vi "Check_Beam_Powers.vi"(3 "Mode":T6, 5 "Traverse line In":T3 {"Row Duration (mins)" format="%#.1f"; "Row No" min=0; "Trace Gas Concentration (%)" min=0.0 format="%#.2f"; "Emission Rate (l/min)" format="%#.2f"; "Tunnel Speed" format="%#.2f"; "Start X" format="%#.2f"; "Start Y" format="%#.2f"; "Start Z" format="%#.2f"; "End X" format="%#.2f"; "End Y" format="%#.2f"; "End Z" format="%#.2f"; "Averaging time (min)" min=0.0 format="%#.1f"}) -> (0 "Error Message":string, 1 "Status":T2, 2 "Traverse line Out":T3 {"Row Duration (mins)" format="%#.1f"; "Row No" min=0; "Trace Gas Concentration (%)" min=0.0 format="%#.2f"; "Emission Rate (l/min)" format="%#.2f"; "Tunnel Speed" format="%#.2f"; "Start X" format="%#.2f"; "Start Y" format="%#.2f"; "Start Z" format="%#.2f"; "End X" format="%#.2f"; "End Y" format="%#.2f"; "End Z" format="%#.2f"; "Averaging time (min)" min=0.0 format="%#.1f"})   [LabVIEW 2010]
uses:
  Gen Trav/Traverse_cluster.ctl
  Gen Trav/Spacing.ctl
  Controls/Multi_run_mode.ctl
  Controls/User_Specific_mode.ctl
  Gen Trav/Multi_Run_Status.ctl
  Controls/Beam_Type.ctl
  ADAM Client/Sub VIs/ADAM Controls/Remember_value_mode.ctl
  Gen Trav/Route mapping/Axis.ctl
  Controls/Save_Data.ctl
  Controls/Setup.ctl
  Globals/Meas_global.vi
  Globals/Constants_global.vi
  Globals/LDA_meas_global_1.vi
  Globals/LDA_meas_global_2.vi
panel:
  out "Light Power":dbl=8.10606551e-08 format="%^#_9e"
  in  "stop":bool
  out "Poor Beam Power?":bool
  in  "Update Datum Powers?":bool
  out "Powers":dbl[](array[numeric]) format="%.4f"
  out "Beam Data":dbl[][](array[numeric]) format="%.4f"
  out "Beam Type":T1 items=["Green Unshifted", "Green Shifted", "Blue Unshifted", "Blue Shifted"]
  # "X                      Y                   Z          Datum Power"
  # "Green Unshifted\nGreen Shifted\nBlue Unshifted\nBlue Shifted"
  # "X           Y            Z"
  # "Start"
  # "End"
  # "X           Y            Z"
  # "Start"
  # "End"
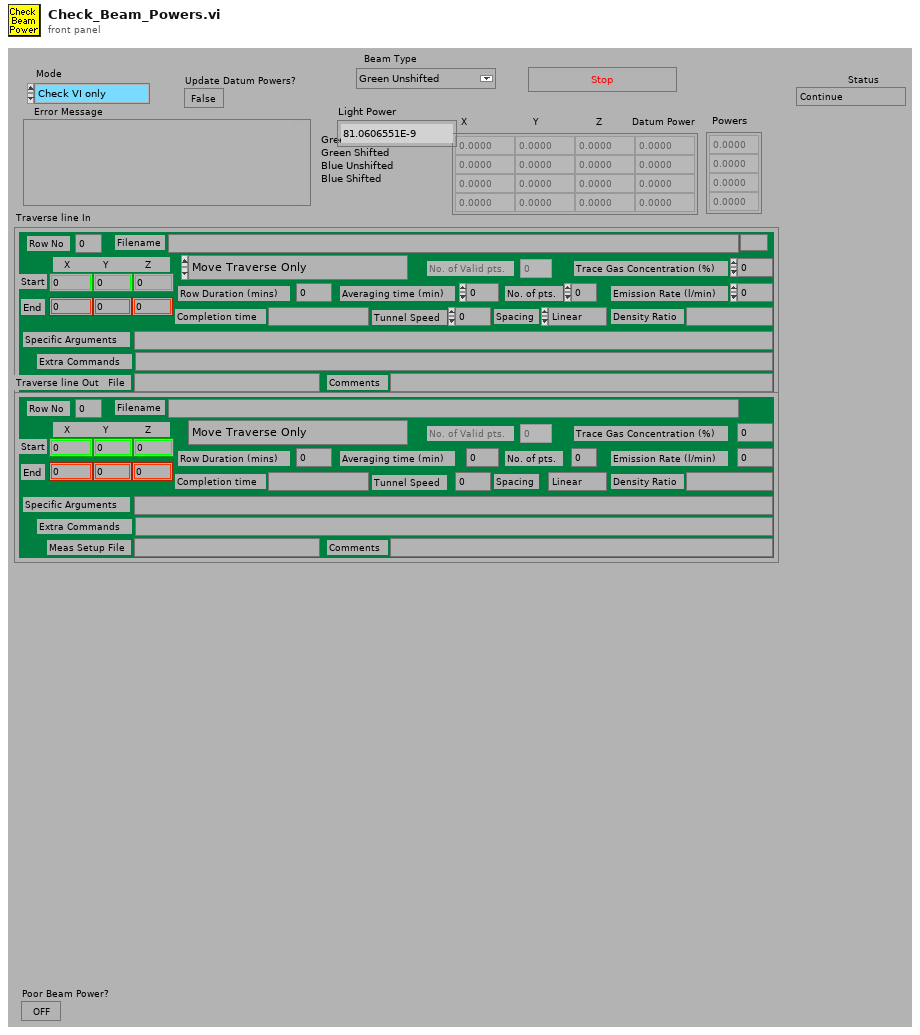
[diagram p1: front panel]
types:
  T1 = typedef "Beam_Type.ctl" = u16
  T2 = typedef "Multi_Run_Status.ctl" = enum16{"Continue", "Jump to Next Point", "Jump to Next Row", "Jump To Fall Back", "Terminate Run"}
  T3 = typedef "Traverse_cluster.ctl" = cluster{"Start X":dbl, "Start Y":dbl, "Start Z":dbl, "End X":dbl, "End Y":dbl, "End Z":dbl, "No. of pts.":i32, "Spacing":T4, "Filename":path, "Tunnel Speed":dbl, "Averaging time (min)":dbl, "Extra Commands":string, "Specific Arguments":string, "Emission Rate (l/min)":dbl, "Trace Gas Concentration (%)":dbl, "Density Ratio":string, "Comments":string, "Row No":i32, "Row Type Selector":T5, "Completion time":string, "Row Duration (mins)":dbl, "No. of Valid pts.":i32, "Meas Setup File":string}
  T4 = typedef "Spacing.ctl" = enum16{"Linear", "Log", "Gauss", "Specified", "N/A"}
  T5 = typedef "Multi_run_mode.ctl" = enum16{"Move Traverse Only", "Set Tunnel Speed Only", "Set Source Only", "Set Measurement Conditions", "Single Measurement", "Vertical Profile", "Lateral Profile", "Longitudinal Profile", "Explore Volume", "Multi-Axis Profile", "Auto Calibrate", "Meas Fast FID Bkgnd", "Check Beam Power", "Scanning Valve Measurement", "Run VI Named:", "Set ADAM Ch", "Wait (minutes)", "Send Message", "Synchronize With:", "Fall Back to this Row", "Turn Off Row Repeating", "Blank Row"}
  T6 = typedef "User_Specific_mode.ctl" = enum16{"Check VI only", "Run VI"}
  T7 = enum32{"Bad", "Idle", "Run top level", "Running"}
  T8 = enum16{"Load From Excel File", "Save to Excel File"}
  T9 = typedef "Remember_value_mode.ctl" = enum16{"Read only", "Read and Write"}
  T10 = typedef "Axis.ctl" = enum16{"X Axis", "X Axis -ve", "Y Axis", "Y Axis -ve", "Z Axis", "Z Axis -ve"}
  T11 = typedef "Save_Data.ctl" = enum16{"Save No Data", "Save Data"}
  T12 = typedef "Setup.ctl" = enum16{"Run Program", "Show Setup", "Save Current Setup", "Setup Front Panel"}
  T13 = typedef "Status_Cluster.ctl" = cluster{"Status":T2, "Error Type":string, "Error Description":string}
  T14 = typedef "BSA_Type.ctl" = enum16{"57N11", "BSA F60"}
  T15 = typedef "BSA_info_Cluster.ctl" = cluster{"GPIB Address":string, "No of Check Bytes":i32, "Extra Info":string, "COLOUR":u32, "Wavelength (nm)":dbl}
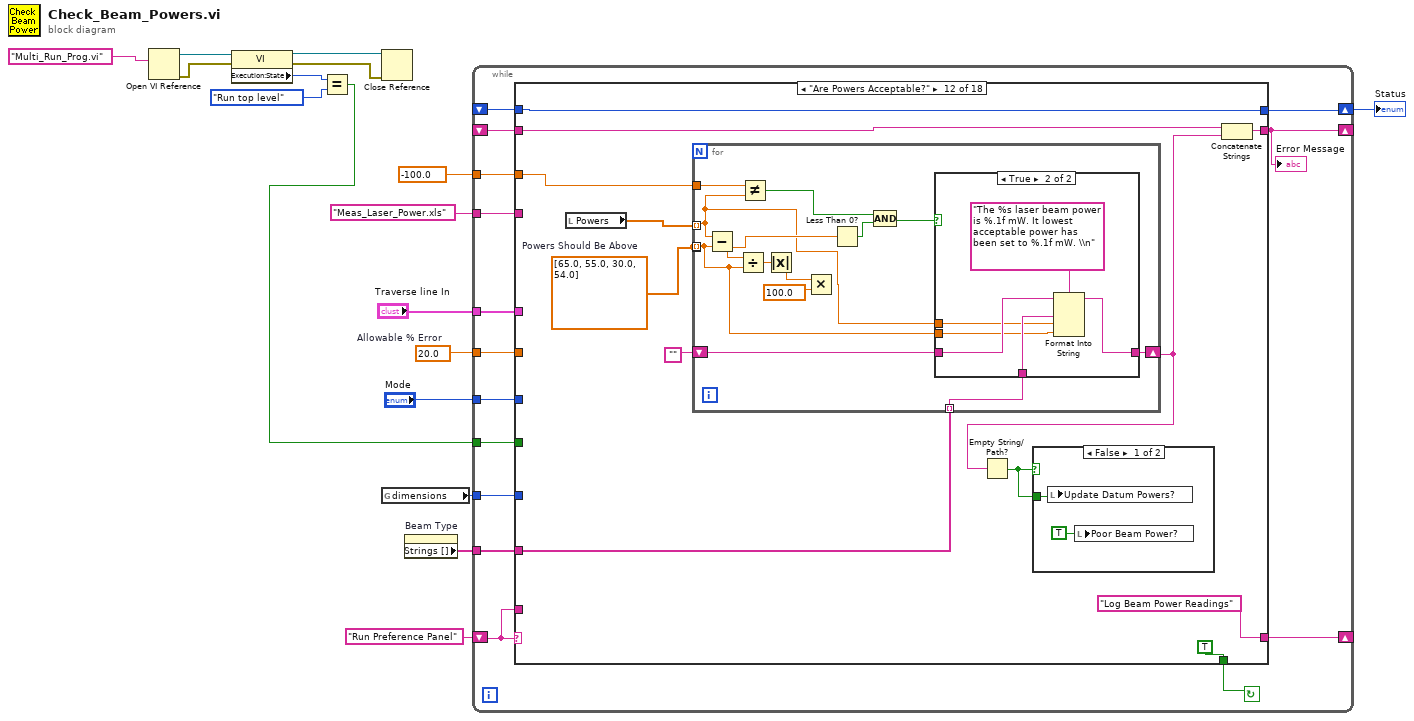
[diagram p0: block diagram]
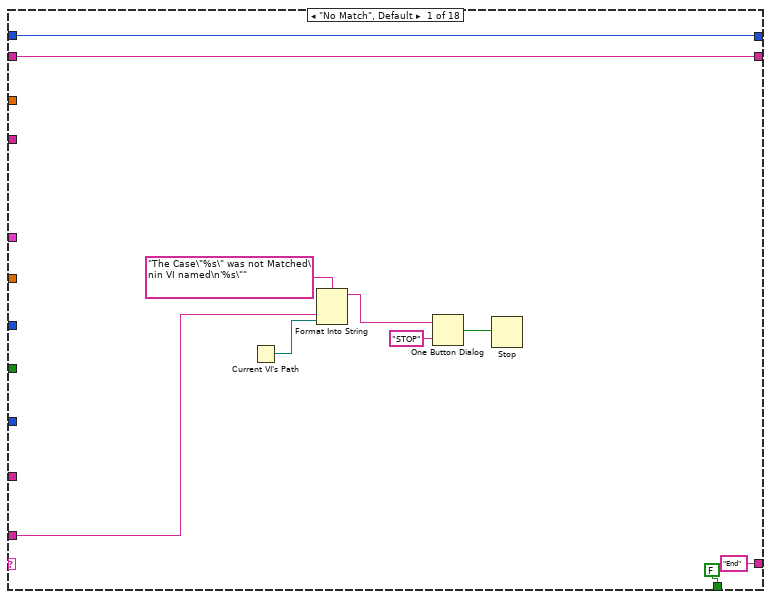
[diagram p2: hidden frame]
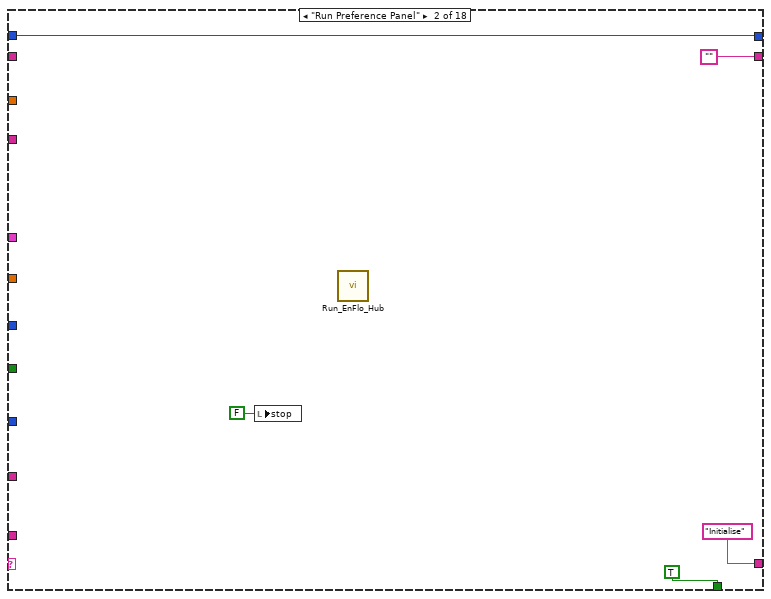
[diagram p3: hidden frame]
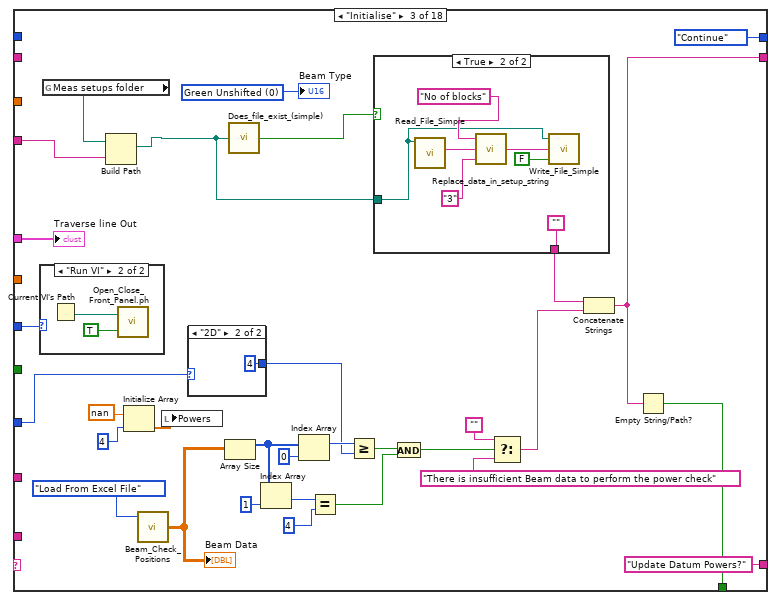
[diagram p4: hidden frame]
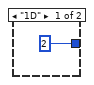
[diagram p5: hidden frame]
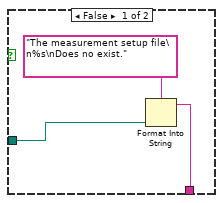
[diagram p6: hidden frame]
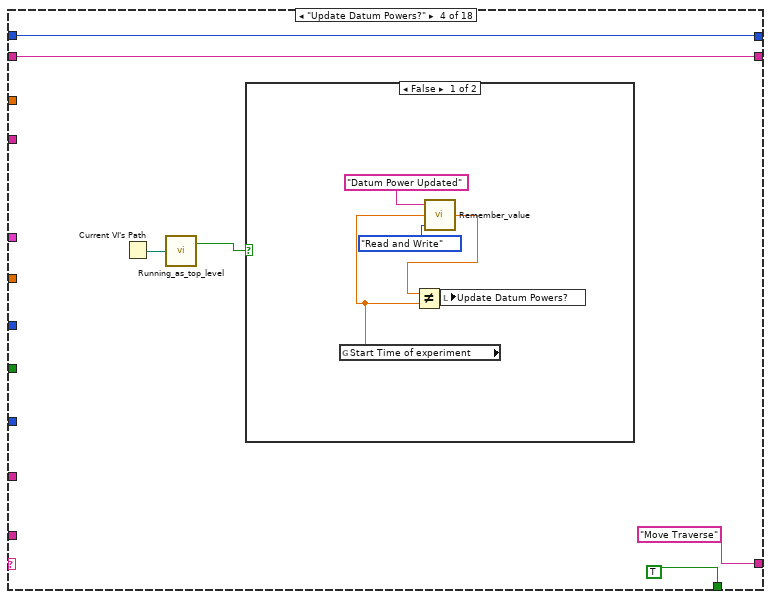
[diagram p8: hidden frame]
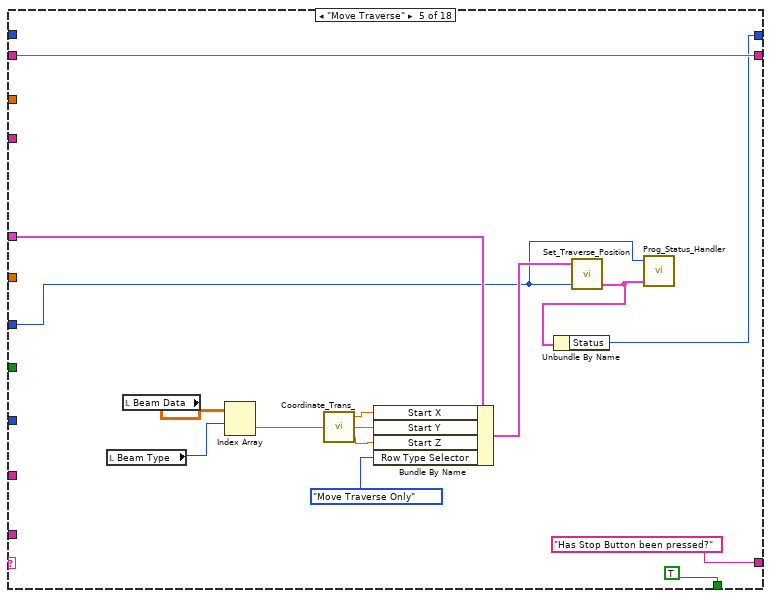
[diagram p10: hidden frame]
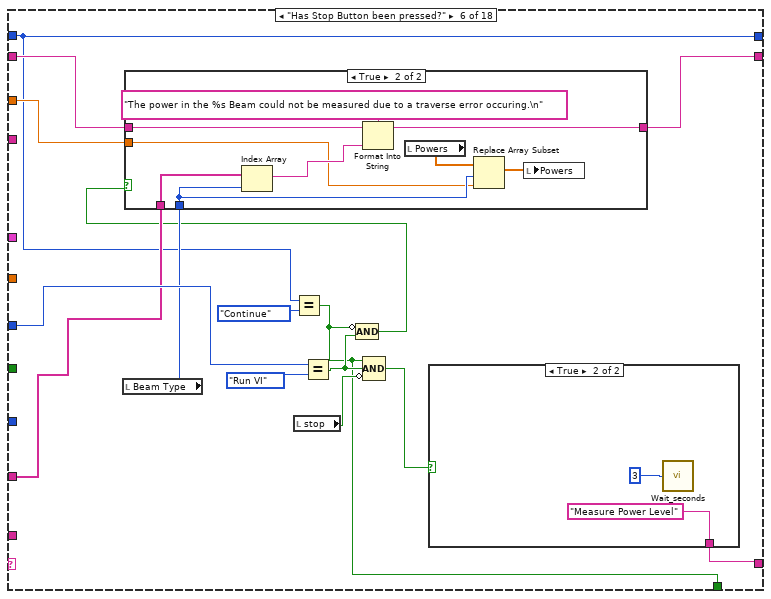
[diagram p11: hidden frame]
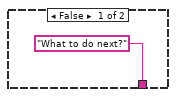
[diagram p13: hidden frame]
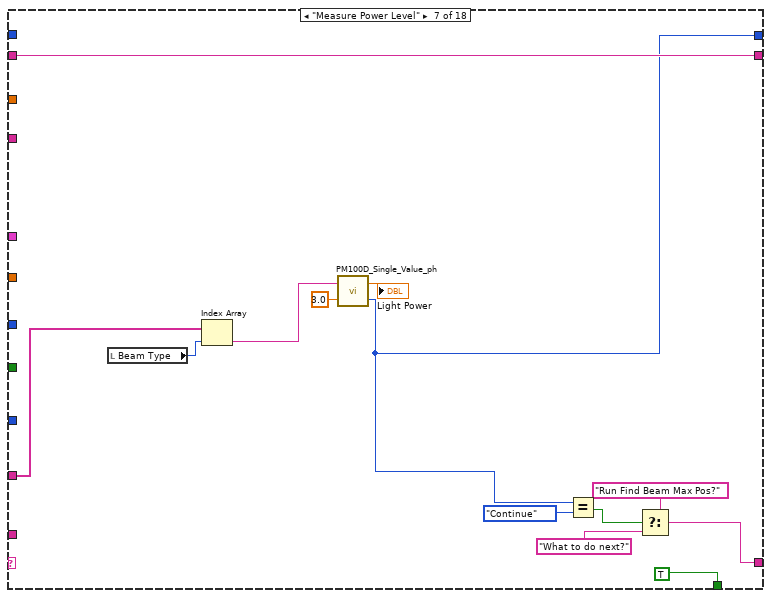
[diagram p14: hidden frame]
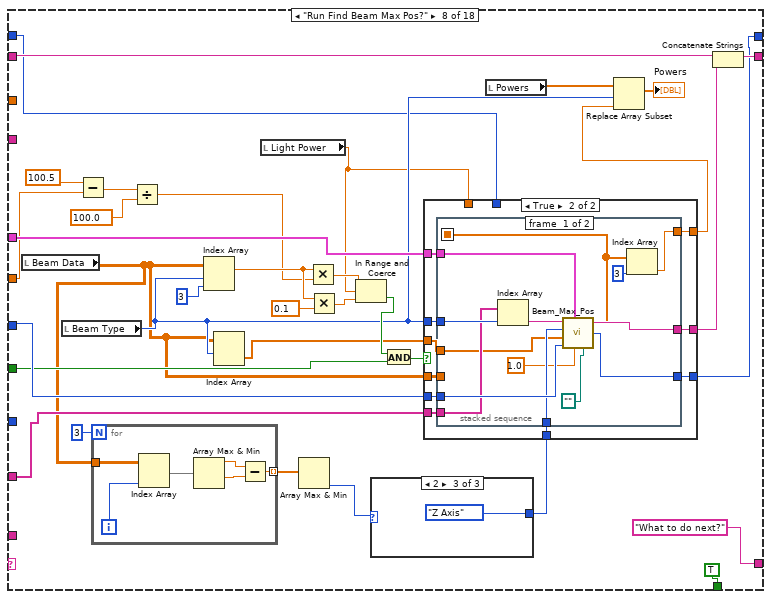
[diagram p15: hidden frame]
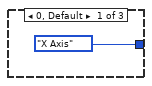
[diagram p16: hidden frame]
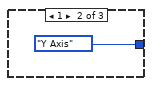
[diagram p17: hidden frame]
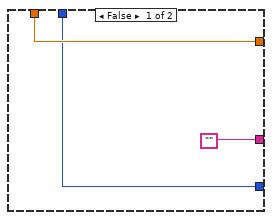
[diagram p18: hidden frame]
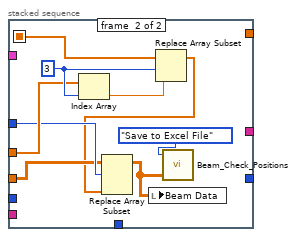
[diagram p19: hidden frame]
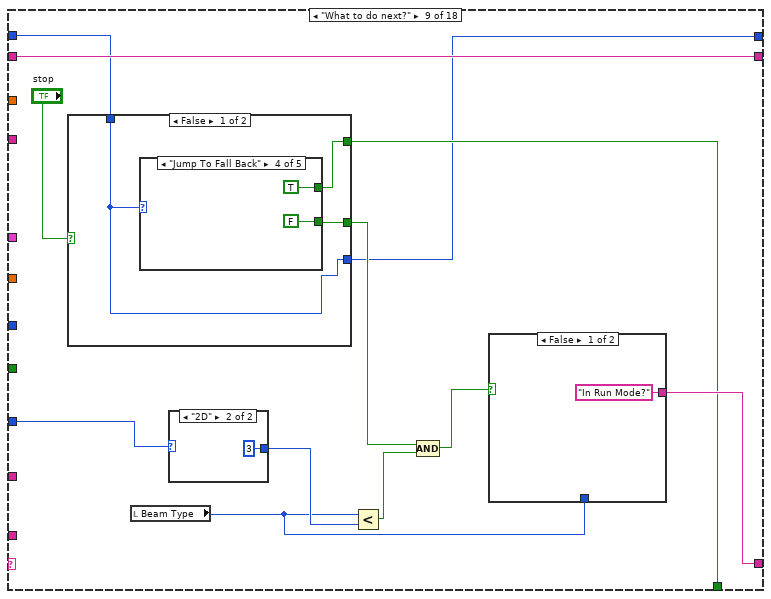
[diagram p20: hidden frame]
diagram:
  w12 = 20.0  # Allowable % Error
  n1 = Open VI Reference(vi path="Multi_Run_Prog.vi") -> (vi reference=w6:refnum<vi>, error out=w7:errorcluster)  [unwired: 1 in, 4 out]
  n2 = property class="VI"(reference=w6, error in=w7) -> (reference out=w8:refnum<vi>, error out=w9:errorcluster, "Execution:State"=w5:T7)
  n3 = Equal?(x=w5, y=T7."Run top level" ("Exec.State")) -> (x = y?=w3:bool)
  n4 = Close Reference(reference=w8, error in (no error)=w9) -> ()  [unwired: 1 out]
  n5 = global read "Meas_global.vi" "dimensions"() -> (w14:enum16{"1D", "2D"})
  n6 = property on="Beam Type" class="Ring (strict)"() -> ("Strings []"=w15:string[])  [unwired: 2 in, 2 out]
  n7 = while {
    tunnel: -100.0 ("Element Data") -> [w21]
    tunnel: w12 -> [w23]
    shift-left: _ -> [w25]
    shift-right: [w24] -> _
    tunnel: "Meas_Laser_Power.xls" -> [w26]
    tunnel: w14 -> [w27]
    tunnel: w15 -> [w30]
    tunnel: "Traverse line In" -> [w31]
    tunnel: "Mode" -> [w32]
    shift-left: "Run Preference Panel" -> [w22]
    shift-right: [w28] -> _
    tunnel: w3 -> [w20]
    shift-right: [w19] -> w1
    shift-left: _ -> [w18]
    stop <- w29 continue-if-true
    n8 = case shown="\"Are Powers Acceptable?\"" w22 {
      tunnel: w31 -> [_ _ w73 _ w118 _ _ w192 _ _ _ _ _ _ _ _ w441 _]
      tunnel: w32 -> [_ _ w70 _ w113 w131 _ w191 _ w280 _ _ _ _ _ _ w445 w450]
      tunnel: w30 -> [_ _ _ _ _ w129 w149 w166 _ _ w293 w335 _ _ _ _ _ _]
      tunnel: [FALSE ("Update Datum Powers?") TRUE ("Update Datum Powers?") w62 TRUE ("Update Datum Powers?") TRUE w120 TRUE TRUE w241 TRUE ("Update Datum Powers?") TRUE TRUE TRUE TRUE ("Update Datum Powers?") TRUE ("Update Datum Powers?") w411 w442 FALSE ("Update Datum Powers?")] -> w29
      tunnel: ["End" "Initialise" "Update Datum Powers?" "Move Traverse" "Has Stop Button been pressed?" w130 w154 "What to do next?" w243 w275 "Are Powers Acceptable?" "Log Beam Power Readings" w362 "Update Datum Powers and Positions" "Take datum velocity measurement?" "Move traverse to datum location" "Take a datum velocity measurement" "End"] -> w28
      tunnel: w27 -> [_ _ w69 _ _ _ _ _ w249 _ _ _ _ _ _ w413 _ _]
      tunnel: w26 -> [_ _ w75 _ _ _ _ _ _ _ _ _ _ _ _ _ _ _]
      tunnel: w25 -> [w34 _ _ w95 w111 w127 w156 w178 w245 w279 w291 w333 w363 w388 w398 w415 w447 w453]
      tunnel: [w34 "" w50 w95 w111 w128 w156 w177 w245 w279 w290 w332 w364 "" w398 w415 w447 w453] -> w24
      tunnel: w23 -> [_ _ _ _ _ _ _ w174 _ _ w286 _ _ _ _ _ _ _]
      tunnel: w22 -> [w37 _ _ _ _ _ _ _ _ _ _ _ _ _ _ _ _ _]
      tunnel: w21 -> [_ _ _ _ _ w126 _ _ _ _ w283 w327 _ _ _ _ _ _]
      tunnel: w20 -> [_ _ _ _ _ _ _ w167 _ _ _ _ _ _ _ w410 _ _]
      tunnel: [w33 w43 Multi_Run_Status."Continue" ("Status") w93 w104 w119 w151 w161 w239 w273 w282 w326 w360 w384 w394 w408 w440 w449] -> w19
      tunnel: w18 -> [w33 w43 _ w93 _ w119 _ w160 w240 w273 w282 w326 w360 w384 w394 w408 _ w448]
      frame "No Match", Default {
        n9 = Current VI's Path() -> (path=w38:path)
        n10 = Format Into String(format string="The Case\"%s\" was not Matched\nin VI named\n'%s\"" ("Format String"), w37, w38) -> (resulting string=w41:string)  [unwired: 2 in, 1 out]
        n11 = One Button Dialog(message=w41, button name ("OK")="STOP") -> (true=w39:bool)
        n12 = Stop(stop? (T)=w39) -> ()
      }
      frame "Run Preference Panel" {
        n13 = local write "stop"(FALSE ("stop")) -> ()
        n14 = call "Run_EnFlo_Hub.vi"() -> ()  [unwired: 8 out]
      }
      frame "Initialise" {
        w77 = T1 0 items=["Green Unshifted", "Green Shifted", "Blue Unshifted", "Blue Shifted"] ("Beam Type")
        n15 = case shown="\"Run VI\"" w70 {
          frame "Check VI only" {
          }
          frame "Run VI" {
            n16 = Current VI's Path() -> (path=w91:path)
            n17 = call "Open_Close_Front_Panel.ph.vi"("Front Panel Window:Open"=TRUE, "VI path"=w91) -> ()  [unwired: 2 out]
          }
        }
        n18 = global read "Constants_global.vi" "Meas setups folder"() -> (w76:path)
        n19 = Build Path(base path=w76, name or relative path=w75) -> (appended path=w51:path)
        n20 = Initialize Array(nan ("Numeric"), 4 ("Dimension Size")) -> (w52:dbl[])
        n21 = call "Beam_Check_Positions.vi"("Mode"=T8."Load From Excel File") -> ("Values Out"=w72:dbl[][])  [unwired: 1 in, 1 out]
        "Beam Data" <- w72
        n22 = local write "Powers"(w52) -> ()
        n23 = case shown="\"2D\"" w69 {
          tunnel: [2 4] -> w67
          frame "1D" {
          }
          frame "2D" {
          }
        }
        n24 = Array Size(array=w72) -> (size(s)=w60:i32[])
        n25 = call "Does_file_exist_(simple).vi"("Pathname"=w51) -> ("exists?"=w74:bool)
        n26 = Index Array(array=w60, index=1 ("Index")) -> (element=w59:i32)
        n27 = Index Array(array=w60, index=0 ("Index")) -> (element=w68:i32)
        n28 = Equal?(x=w59, y=4) -> (x = y?=w56:bool)
        n29 = Greater Or Equal?(x=w68, y=w67) -> (x >= y?=w57:bool)
        n30 = case shown="True" w74 {
          tunnel: w51 -> [w83 w84]
          tunnel: [w81 ""] -> w64
          frame False {
            n31 = Format Into String(format string="The measurement setup file\n%s\nDoes no exist." ("Format String"), w83) -> (resulting string=w81:string)  [unwired: 2 in, 1 out]
          }
          frame True {
            n32 = call "Read_File_Simple.vi"("Filename"=w84) -> ("string"=w89:string)  [unwired: 2 in, 7 out]
            n33 = call "Replace_data_in_setup_string.vi"("New data string"="3", "Input string"=w89, "Variable name"="No of blocks") -> ("Appended string"=w86:string)
            n34 = call "Write_File_Simple.vi"("append to file? (new file:F)"=FALSE, "character string"=w86, "file path"=w84) -> ()  [unwired: 2 out]
          }
        }
        n35 = And(x=w57, y=w56) -> (x .and. y?=w55:bool)
        n36 = Select(t="", s=w55, f="There is insufficient Beam data to perform the power check") -> (s? t:f=w63:string)
        n37 = Concatenate Strings(w64, w63) -> (w50:string)
        n38 = Empty String/Path?(string/path=w50) -> (empty?=w62:bool)
        "Beam Type" <- w77
        "Traverse line Out" <- w73
      }
      frame "Update Datum Powers?" {
        n39 = Current VI's Path() -> (path=w97:path)
        n40 = call "Running_as_top_level.vi"("Vi path name"=w97) -> ("Top Level"=w96:bool)  [unwired: 1 out]
        n41 = case shown="False" w96 {
          frame False {
            n42 = global read "Meas_global.vi" "Start Time of experiment"() -> (w101:dbl)
            n43 = call "Remember_value.vi"("Mode"=Remember_value_mode."Read and Write", "Input Value"=w101, "Ch name"="Datum Power Updated") -> ("Output Value"=w102:dbl)
            n44 = Not Equal?(x=w102, y=w101) -> (x != y?=w99:bool)
            n45 = local write "Update Datum Powers?"(w99) -> ()
          }
          frame True {
          }
        }
      }
      frame "Move Traverse" {
        n46 = local read "Beam Type"() -> (w109:T1)
        n47 = local read "Beam Data"() -> (w110:dbl[][])
        n48 = Index Array(array=w110, index (row)=w109) -> (element=w105:dbl[])  [unwired: 1 in]
        n49 = call "Coordinate_Trans_.vi"("Input Position"=w105) -> ("X"=w108:dbl, "Y"=w107:dbl, "Z"=w106:dbl)
        n50 = Bundle By Name(cluster=w118, "Start X"=w108, "Start Y"=w107, "Start Z"=w106, "Row Type Selector"=Multi_run_mode."Move Traverse Only") -> (w116:T3)
        n51 = call "Set_Traverse_Position.vi"("Simulate/Run"=w113, "Traverse line"=w116) -> ("Status Cluster"=w114:T13)  [unwired: 1 in, 2 out]
        n52 = Unbundle By Name(w114) -> ("Status"=w104:T2)
        n53 = call "Prog_Status_Handler.vi"("Status Cluster"=w114, "Simulate/Run"=w113) -> ()  [unwired: 2 out]
      }
      frame "Has Stop Button been pressed?" {
        n54 = local read "Beam Type"() -> (w125:T1)
        n55 = Equal?(x=w119, y=Multi_Run_Status."Continue" ("Status")) -> (x = y?=w120:bool)
        n56 = local read "stop"() -> (w124:bool)
        n57 = Equal?(x=w131, y=User_Specific_mode."Run VI" ("Mode")) -> (x = y?=w122:bool)
        n58 = Compound Arithmetic op=AND(invert w120, w122) -> (w121:bool)
        n59 = case shown="True" w121 {
          tunnel: w125 -> [_ w136]
          tunnel: w129 -> [_ w143]
          tunnel: w127 -> [w134 w140]
          tunnel: [w134 w139] -> w128
          tunnel: w126 -> [_ w135]
          frame False {
          }
          frame True {
            n60 = Index Array(array=w143, index=w136) -> (element=w142:string)
            n61 = Format Into String(format string="The power in the %s Beam could not be measured due to a traverse error occuring.\n" ("Format String"), initial string=w140, w142) -> (resulting string=w139:string)  [unwired: 1 in, 1 out]
            n62 = local read "Powers"() -> (w138:dbl[])
            n63 = Replace Array Subset(array=w138, new element=w135, index=w136) -> (w137:dbl[])
            n64 = local write "Powers"(w137) -> ()
          }
        }
        n65 = Compound Arithmetic op=AND(w120, w122, invert w124) -> (w123:bool)
        n66 = case shown="True" w123 {
          tunnel: ["What to do next?" "Measure Power Level"] -> w130
          frame False {
          }
          frame True {
            n67 = call "Wait_seconds.vi"("Seconds to wait"=u32 3) -> ()
          }
        }
      }
      frame "Measure Power Level" {
        n68 = local read "Beam Type"() -> (w150:T1)
        n69 = Index Array(array=w149, index=w150) -> (element=w148:string)
        n70 = call "PM100D_Single_Value_ph.vi"("Averaging Period (s)"=3.0, "Beam Name"=w148) -> ("Status"=w151:T2, "Light Power mW"=→"Light Power":dbl)
        n71 = Equal?(x=w151, y=Multi_Run_Status."Continue" ("Status")) -> (x = y?=w157:bool)
        n72 = Select(t="Run Find Beam Max Pos?", s=w157, f="What to do next?") -> (s? t:f=w154:string)
      }
      frame "Run Find Beam Max Pos?" {
        n73 = local read "Beam Data"() -> (w163:dbl[][])
        n74 = local read "Beam Type"() -> (w165:T1)
        n75 = Subtract(x=100.5, y=w174) -> (x-y=w173:dbl)
        n76 = for {
          N: 3 -> [_]
          tunnel: w163 -> [w201]
          tunnel: [w197] -> w189 mode=indexing
          i -> [w202]
          n77 = Index Array(array=w201, index (col)=w202) -> (element=w200:dbl[])  [unwired: 1 in]
          n78 = Array Max & Min(array=w200) -> (max value=w199:dbl, min value=w198:dbl)  [unwired: 2 out]
          n79 = Subtract(x=w199, y=w198) -> (x-y=w197:dbl)
        }
        n80 = Divide(x=w173, y=100.0) -> (x/y=w171:dbl)
        n81 = Index Array(array=w163, index (row)=w165, index (col)=3 ("Index")) -> (element=w185:dbl)
        n82 = Index Array(array=w163, index (row)=w165) -> (element=w164:dbl[])  [unwired: 1 in]
        n83 = local read "Light Power"() -> (w162:dbl)
        n84 = Array Max & Min(array=w189) -> (min index (indices)=w188:i32)  [unwired: 3 out]
        n85 = Multiply(x=w185, y=w171) -> (x*y=w183:dbl)
        n86 = Multiply(x=w185, y=0.1) -> (x*y=w182:dbl)
        n87 = In Range and Coerce(upper limit=w183, x=w162, lower limit=w182) -> (In Range?=w169:bool)  [unwired: 1 out]
        n88 = case shown="2" w188 {
          tunnel: [Axis."X Axis" ("Fixed Axis") Axis."Y Axis" ("Fixed Axis") Axis."Z Axis" ("Fixed Axis")] -> w187
          frame 0, Default {
          }
          frame 1 {
          }
          frame 2 {
          }
        }
        n89 = And(x=w169, y=w167) -> (x .and. y?=w168:bool)
        n90 = case shown="True" w168 {
          tunnel: w165 -> [_ w210]
          tunnel: w192 -> [_ w215]
          tunnel: w191 -> [_ w214]
          tunnel: w187 -> [_ w213]
          tunnel: [w205 w212] -> w179
          tunnel: w162 -> [w205 _]
          tunnel: ["" w211] -> w176
          tunnel: w166 -> [_ w209]
          tunnel: w164 -> [_ w208]
          tunnel: w163 -> [_ w207]
          tunnel: [w203 w206] -> w161
          tunnel: w160 -> [w203 _]
          frame False {
          }
          frame True {
            n91 = stacked-sequence {
              seq-local: [w218 _] -> [_ w236]
              tunnel: w215 -> [w229 _]
              tunnel: w214 -> [w228 _]
              tunnel: w213 -> [w227 _]
              tunnel: [w225 _] -> w212
              tunnel: [w224 _] -> w211
              tunnel: w210 -> [w222 w234]
              tunnel: w209 -> [w221 _]
              tunnel: w208 -> [w219 w235]
              tunnel: w207 -> [_ w233]
              tunnel: [w216 _] -> w206
              frame #0 {
                n92 = Index Array(array=w221, index=w222) -> (element=w220:string)
                n93 = call "Beam_Max_Pos.vi"("Picture Log"=path "", "Search Step (mm)"=1.0, "Mode"=w228, "Starting Position"=w219, "Traverse line In"=w229, "Fixed Axis"=w227, "Beam Name"=w220) -> ("Status"=w216:T2, "Beam maxima"=w218:dbl[], "Message"=w224:string)  [unwired: 1 out]
                n94 = Index Array(array=w218, index=3 ("Index")) -> (element=w225:dbl)
              }
              frame #1 {
                w237 = 3 ("index")
                n95 = Index Array(array=w235, index=w237) -> (element=w238:dbl)
                n96 = Replace Array Subset(array=w236, new element=w238, index=w237) -> (w230:dbl[])
                n97 = Replace Array Subset(array=w233, new element=w230, index (row)=w234) -> (w232:dbl[][])  [unwired: 1 in]
                n98 = local write "Beam Data"(w232) -> ()
                n99 = call "Beam_Check_Positions.vi"("Values"=w232, "Mode"=T8."Save to Excel File") -> ()  [unwired: 2 out]
              }
            }
          }
        }
        n100 = local read "Powers"() -> (w181:dbl[])
        n101 = Replace Array Subset(array=w181, new element=w179, index=w165) -> (→"Powers":dbl[])
        n102 = Concatenate Strings(w178, w176) -> (w177:string)
      }
      frame "What to do next?" {
        n103 = case shown="False" "stop" {
          tunnel: [w253 FALSE] -> w242
          tunnel: [w252 FALSE] -> w241
          tunnel: w240 -> [w251 _]
          tunnel: [w251 Multi_Run_Status."Terminate Run" ("Status")] -> w239
          frame False {
            n104 = case shown="\"Jump To Fall Back\"" w251 {
              tunnel: [TRUE TRUE FALSE FALSE FALSE] -> w253
              tunnel: [TRUE TRUE TRUE TRUE FALSE] -> w252
              frame "Continue" {
              }
              frame "Jump to Next Point" {
              }
              frame "Jump to Next Row" {
              }
              frame "Jump To Fall Back" {
              }
              frame "Terminate Run" {
              }
            }
          }
          frame True {
          }
        }
        n105 = local read "Beam Type"() -> (w246:T1)
        n106 = case shown="\"2D\"" w249 {
          tunnel: [1 3] -> w250
          frame "1D" {
          }
          frame "2D" {
          }
        }
        n107 = Less?(x=w246, y=w250) -> (x < y?=w248:bool)
        n108 = Compound Arithmetic op=AND(w242, w248) -> (w247:bool)
        n109 = case shown="False" w247 {
          tunnel: w246 -> [_ w270]
          tunnel: ["In Run Mode?" "Move Traverse"] -> w243
          frame False {
          }
          frame True {
            n110 = Increment(x=w270) -> (x+1=w269:T1)
            n111 = local write "Beam Type"(w269) -> ()
          }
        }
      }
      frame "In Run Mode?" {
        n112 = Equal?(x=w280, y=User_Specific_mode."Run VI" ("Mode")) -> (x = y?=w277:bool)
        n113 = Select(t="Compare Powers with Datum values", s=w277, f="Move traverse to datum location") -> (s? t:f=w275:string)
      }
      frame "Compare Powers with Datum values" {
        n114 = local read "Beam Data"() -> (w296:dbl[][])
        n115 = local read "Powers"() -> (w295:dbl[])
        n116 = Index Array(array=w296, index (col)=3 ("Index")) -> (element=w294:dbl[])  [unwired: 1 in]
        n117 = for {
          tunnel: w295 -> [w301] mode=indexing
          tunnel: w294 -> [_] mode=indexing
          tunnel: w294 -> [w312] mode=indexing
          shift-right: [w316] -> w289
          shift-left: "" -> [w318]
          tunnel: w293 -> [w317] mode=indexing
          tunnel: "Update Datum Powers?" -> [w315]
          tunnel: w286 -> [w302]
          tunnel: w283 -> [w300]
          n118 = Subtract(x=w301, y=w312) -> (x-y=w310:dbl)
          n119 = Not Equal?(x=w300, y=w301) -> (x != y?=w299:bool)
          n120 = Divide(x=w310, y=w312) -> (x/y=w311:dbl)
          n121 = Greater Than 0?(x=w310) -> (x > 0?=w306:bool)
          n122 = Absolute Value(x=w311) -> (abs(x)=w309:dbl)
          n123 = Multiply(x=w309, y=100.0) -> (x*y=w307:dbl)
          n124 = Greater?(x=w307, y=w302) -> (0:w308:bool)
          n125 = Select(t="above", s=w306, f="below") -> (s? t:f=w303:string)
          n126 = Compound Arithmetic op=AND(w299, invert w315, w308) -> (w314:bool)
          n127 = case shown="True" w314 {
            tunnel: w318 -> [w319 w324]
            tunnel: w317 -> [_ w325]
            tunnel: [w319 w323] -> w316
            tunnel: w307 -> [_ w321]
            tunnel: w303 -> [_ w320]
            frame False {
            }
            frame True {
              n128 = Format Into String(format string="The %s laser beam is %.1f%% %s its datum value\\n" ("Format String"), initial string=w324, w325, w321, w320) -> (resulting string=w323:string)  [unwired: 1 in, 1 out]
            }
          }
        }
        n129 = Empty String/Path?(string/path=w289) -> (empty?=w288:bool)
        n130 = Not(x=w288) -> (.not. x?=→"Poor Beam Power?":bool)
        n131 = Concatenate Strings(w291, w289) -> (w290:string)
      }
      frame "Are Powers Acceptable?" {
        w330 = dbl[] [65.0, 55.0, 30.0, 54.0]  # Powers Should Be Above
        n132 = local read "Powers"() -> (w336:dbl[])
        n133 = for {
          tunnel: w336 -> [w341] mode=indexing
          tunnel: w330 -> [_] mode=indexing
          tunnel: w330 -> [w340] mode=indexing
          shift-right: [w350] -> w331
          shift-left: "" -> [w352]
          tunnel: w335 -> [w351] mode=indexing
          tunnel: w327 -> [w345]
          n134 = Subtract(x=w341, y=w340) -> (x-y=w346:dbl)
          n135 = Divide(x=w346, y=w340) -> (x/y=w348:dbl)
          n136 = Not Equal?(x=w345, y=w341) -> (x != y?=w342:bool)
          n137 = Absolute Value(x=w348) -> (abs(x)=w347:dbl)
          n138 = Multiply(x=w347, y=100.0) -> ()  [unwired: 1 out]
          n139 = Less Than 0?(x=w346) -> (x < 0?=w343:bool)
          n140 = Compound Arithmetic op=AND(w342, w343) -> (w344:bool)
          n141 = case shown="True" w344 {
            tunnel: w352 -> [w353 w358]
            tunnel: w351 -> [_ w359]
            tunnel: [w353 w357] -> w350
            tunnel: w341 -> [_ w355]
            tunnel: w340 -> [_ w354]
            frame False {
            }
            frame True {
              n142 = Format Into String(format string="The %s laser beam power is %.1f mW. It lowest acceptable power has been set to %.1f mW. \\n" ("Format String"), initial string=w358, w359, w355, w354) -> (resulting string=w357:string)  [unwired: 1 in, 1 out]
            }
          }
        }
        n143 = Empty String/Path?(string/path=w331) -> (empty?=w329:bool)
        n144 = case shown="False" w329 {
          tunnel: w329 -> [w339 _]
          frame False {
            n145 = local write "Update Datum Powers?"(w339) -> ()
            n146 = local write "Poor Beam Power?"(TRUE ("Poor Beam Power?")) -> ()
          }
          frame True {
          }
        }
        n147 = Concatenate Strings(w333, w331) -> (w332:string)
      }
      frame "Log Beam Power Readings" {
        n148 = local read "Poor Beam Power?"() -> (w365:bool)
        n149 = local read "Beam Data"() -> (w368:dbl[][])
        n150 = local read "Powers"() -> (w367:dbl[])
        n151 = case shown="True" w365 {
          tunnel: w363 -> [w374 w378]
          tunnel: [w374 w376] -> w364
          tunnel: [w373 w375] -> w362
          tunnel: "Send Error Email" ("f") -> [w370 w375]
          frame False {
            n152 = Empty String/Path?(string/path=w374) -> (empty?=w371:bool)
            n153 = Select(t="Update Datum Powers and Positions", s=w371, f=w370) -> (s? t:f=w373:string)
          }
          frame True {
            n154 = Concatenate Strings(w378, "Please come and check the system As Soon As Possible!\nThe probe may have collided with something or the optical fibres could be getting damaged due to poor launch efficiency! £18,000 TO REPAIR!!\nThe Multi Run will continue." ("Substring")) -> (w376:string)
          }
        }
        n155 = for {
          tunnel: w368 -> [w383] mode=indexing
          tunnel: w367 -> [w380] mode=indexing
          tunnel: [w379] -> w366 mode=indexing
          n156 = Array Subset(array=w383, length=3 ("Array Length")) -> (w381:dbl[])  [unwired: 1 in]
          n157 = Build Array (concatenate)(w381, w380) -> (w379:dbl[])
        }
        n158 = call "Log_beam_power.vi"("Message"=w363, "Beam Data"=w366) -> ()  [unwired: 4 out]
      }
      frame "Send Error Email" {
        w392 = FALSE  # Dialog Box (T)
        n159 = Bundle By Name(cluster=errorcluster {"status"=FALSE, "code"=0, "source"=""} ("error in (no error)"), "source"=w388, "status"=TRUE ("Bundle Element")) -> (w390:errorcluster)
        n160 = call "EnFlo_Error_Handler.vi"("error in (no error)"=w390, "Error Type"="Beam Power", "Dialog Box (T)"=w392) -> ()  [unwired: 3 out]
      }
      frame "Update Datum Powers and Positions" {
        n161 = local read "Update Datum Powers?"() -> (w395:bool)
        n162 = case shown="True" w395 {
          frame False {
          }
          frame True {
            n163 = local read "Beam Data"() -> (w401:dbl[][])
            n164 = local read "Powers"() -> (w399:dbl[])
            n165 = for {
              tunnel: w401 -> [w407] mode=indexing
              tunnel: [w404] -> w400 mode=indexing
              tunnel: w399 -> [w403] mode=indexing
              n166 = Array Subset(array=w407, length=3 ("Array Length")) -> (w405:dbl[])  [unwired: 1 in]
              n167 = Build Array (concatenate)(w405, w403) -> (w404:dbl[])
            }
            n168 = call "Beam_Check_Positions.vi"("Values"=w400, "Mode"=T8."Save to Excel File") -> ()  [unwired: 2 out]
          }
        }
      }
      frame "Take datum velocity measurement?" {
        n169 = global read "LDA_meas_global_1.vi" "BSA Type"() -> (w409:T14)
        n170 = case shown="\"57N11\"" w409 {
          tunnel: w413 -> [w418 _]
          tunnel: [w417 TRUE] -> w412
          tunnel: w410 -> [w416 _]
          frame "57N11" {
            n171 = stacked-sequence {
              tunnel: w418 -> [_ w431]
              tunnel: [_ w427] -> w417
              tunnel: w416 -> [w419 _]
              frame #0 {
                n172 = case shown="True" w419 {
                  frame False {
                  }
                  frame True {
                    n173 = stacked-sequence {
                      frame #0 {
                        n174 = global read "LDA_meas_global_2.vi" "BSA2 info"() -> (w420:T15)
                        n175 = global read "LDA_meas_global_1.vi" "BSA1 info"() -> (w425:T15)
                        n176 = Unbundle By Name(w420) -> ("GPIB Address"=w421:string)
                        n177 = Unbundle By Name(w425) -> ("GPIB Address"=w424:string)
                        n178 = call "Set_BSA_voltage_On_Off.vi"("GPIB address"=w421, "High Voltage"=TRUE) -> ()  [unwired: 1 in, 5 out]
                        n179 = call "Set_BSA_voltage_On_Off.vi"("GPIB address"=w424, "High Voltage"=TRUE) -> ()  [unwired: 1 in, 5 out]
                      }
                      frame #1 {
                        n180 = call "Wait_seconds.vi"("Seconds to wait"=u32 5) -> ()
                      }
                    }
                  }
                }
              }
              frame #1 {
                w428 = 7.0 ("y")
                n181 = call "LDA_data_rate.vi"() -> ("Data rate (Hz) BSA1"=w432:dbl, "Data rate (Hz) BSA2"=w429:dbl)  [unwired: 1 out]
                n182 = Greater?(x=w432, y=w428) -> (0:w430:bool)
                n183 = case shown="\"1D\"" w431 {
                  tunnel: w430 -> [w433 w437]
                  tunnel: w429 -> [_ w436]
                  tunnel: w428 -> [_ w435]
                  tunnel: [w433 w434] -> w427
                  frame "1D" {
                  }
                  frame "2D" {
                    n184 = Greater?(x=w436, y=w435) -> (0:w438:bool)
                    n185 = And(x=w437, y=w438) -> (x .and. y?=w434:bool)
                  }
                }
              }
            }
          }
          frame "BSA F60" {
          }
        }
        n186 = And(x=w412, y=w410) -> (x .and. y?=w411:bool)
      }
      frame "Move traverse to datum location" {
        n187 = call "Set_Traverse_Position.vi"("Simulate/Run"=w445, "Traverse line"=w441) -> ("Status Cluster"=w444:T13)  [unwired: 1 in, 2 out]
        n188 = Unbundle By Name(w444) -> ("Status"=w440:T2)
        n189 = Equal?(x=Multi_Run_Status."Continue" ("Status"), y=w440) -> (x = y?=w442:bool)
      }
      frame "Take a datum velocity measurement" {
        n190 = case shown="\"Run VI\"" w450 {
          tunnel: [w454 w455] -> w449
          tunnel: w448 -> [w454 _]
          frame "Check VI only" {
          }
          frame "Run VI" {
            n191 = flat-sequence {
              tunnel: [w460] -> w457
              tunnel: [w459] -> w456
              tunnel: [w458] -> w455
              tunnel: w457 -> [w469]
              tunnel: w456 -> [w468]
              frame #0 {
                w462 = 1.0  # Averaging time (min)
                w465 = FALSE  # Acquisition Interlock
                w466 = FALSE  # Open Front Panel
                w467 = FALSE  # Remote control
                n192 = call "Create_Error_log_folders.vi"("Log Filename"="LDA_Datum_Vel.xls" ("Input Element")) -> ("Server copy Location"=w459:path, "Local Log File"=w460:path)  [unwired: 2 in, 1 out]
                n193 = call "Code_to_run.vi"("Open Front Panel"=w466, "Acquisition Interlock"=w465, "setup"=Setup."Run Program", "Remote control"=w467, "File"=Save_Data."Save Data", "Results Filename"=w460, "Averaging time (min)"=w462) -> ("Status"=w458:T2)  [unwired: 4 in, 4 out]
              }
              frame #1 {
                n194 = call "Updated_File_Copy.vi"("Target Path"=w468, "Source Path"=w469) -> ()  [unwired: 2 out]
              }
            }
          }
        }
      }
    }
    "Error Message" <- w24
  }
  "Status" <- w1
